vi "23384_Davis_Poku_Amankwa_Amankwa.DavisPoku.MNE1201.4.5_348257_1447324650.vi"() -> ()   [LabVIEW 2018]
uses:
  <vilib>/imath/engines/lvmath2/RunTimeEngine/Managers/WorkSpace/UID Generator.vi
  <vilib>/imath/engines/lvmath2/RunTimeEngine/RunTimeType/NIMS_RunTimeType_From StrictType (excl LVString).vi
  <instcachedir>/0/NIMS_RunTimeType_From StrictType (excl LVString)_E7E34A65C99947108168652BAD14964D.lvgen/NIMS_RunTimeType_From StrictType (excl LVString)_E7E34A65C99947108168652BAD14964D_000.vi
  <vilib>/imath/engines/lvmath2/RunTimeEngine/LocalVariableDefStatement/MC_LocalVariableDefStatement_Display.vi
  <vilib>/imath/engines/lvmath2/RunTimeEngine/BuiltInFunctions/quadn_trap/NIMS_quadn_trap(GV,GV).vi
  <instcachedir>/0/NIMS_quadn_trap(GV,GV)_ED679A1DCACA4B2C9F69518D213B3EC5.lvgen/NIMS_quadn_trap(GV,GV)_ED679A1DCACA4B2C9F69518D213B3EC5_000.vi
  <vilib>/imath/engines/lvmath2/RunTimeEngine/ErrorHandling/NIMS_Error From Error Code.vi
  <vilib>/imath/engines/lvmath2/RunTimeEngine/Managers/SymbolTable/Clear UID.vi
  <vilib>/imath/engines/lvmath2/RunTimeEngine/NodeEndStatement/NIMS_NodeEndStatement_Output.vi
  <instcachedir>/0/NIMS_NodeEndStatement_Output_53EC0D466D134D7ABD903AC30B43404B.lvgen/NIMS_NodeEndStatement_Output_53EC0D466D134D7ABD903AC30B43404B_001.vi
  <vilib>/imath/engines/lvmath2/RunTimeEngine/ErrorHandling/NIMS_Finalize Error.vi
  <vilib>/imath/engines/lvmath2/RunTimeEngine/Managers/SymbolTable/NIMS_WorkSpace.lvlib
panel:
  out "For you to achieve precision to 5 decimal places then the values of x between 0 and 1 has to be 50":dbl
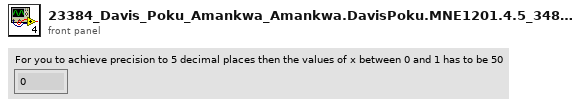
[diagram p1: front panel]
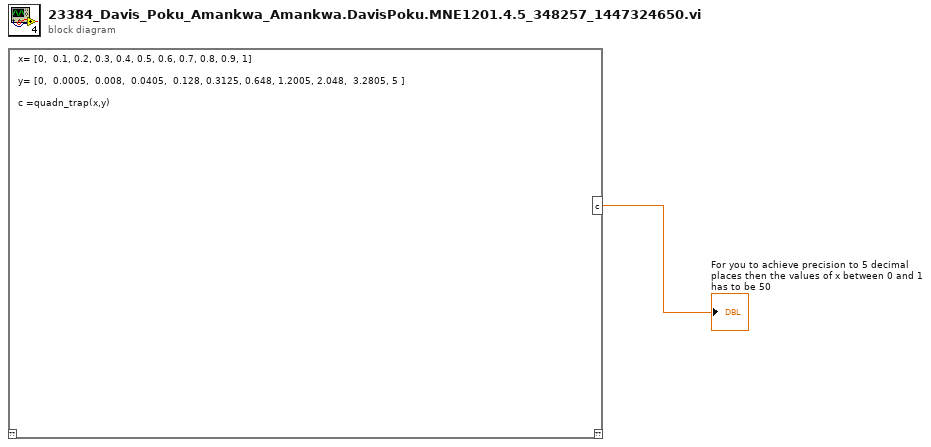
[diagram p0: block diagram]
diagram:
  n1 = mathscript code="x= [0,  0.1, 0.2, 0.3, 0.4, 0.5, 0.6, 0.7, 0.8, 0.9, 1]\n\ny= [0,  0.0005,  0.008,  0.0405,  0.128, 0.3125, 0.648, 1.2005, 2.048,  3.2805, 5 ]\n\nc =quadn_trap(x,y)"() -> ("c"=→"For you to achieve precision to 5 decimal places then the values of x between 0 and 1 has to be 50":dbl)  [unwired: 1 in, 1 out]
